vi "waitForCommandId.vi"(8 "error in (no error)":errorcluster, 11 "M1M3SAL in":refnum<class "M1M3SAL.lvclass">) -> (0 "error out":errorcluster, 2 "CommandId":T1, 3 "M1M3SAL out":refnum<class "M1M3SAL.lvclass">)   [LabVIEW 2016, in "M1M3SupportCommunicator.lvlib" / "M1M3SAL.lvclass"]
uses:
  M1M3SAL.lvclass
  DataTypes/Topics/Parts/CommandId.ctl
  M1M3SAL.lvclass/M1M3SAL.ctl
  UserEvents/UserEvents.lvclass/UserEvents.ctl
  UserEvents/UserEvents.lvclass
  DataTypes/Topics/M1M3SupportTopics.lvlib
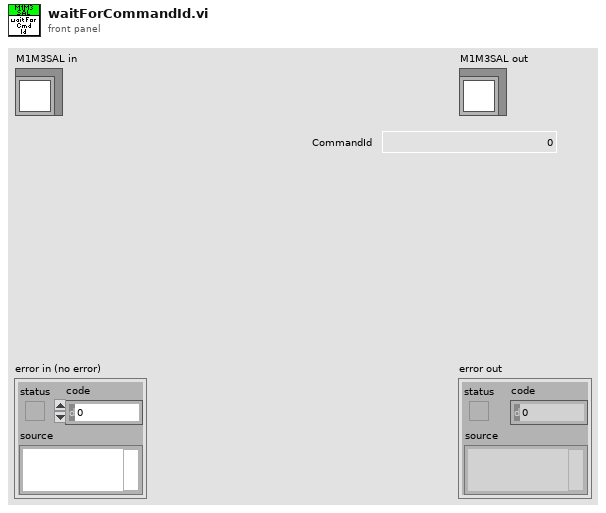
[diagram p1: front panel]
types:
  T1 = typedef "M1M3SupportTopics.lvlib/CommandId.ctl" = i32
  T2 = typedef "M1M3Communicator.lvlib/CommandId.ctl" = i32
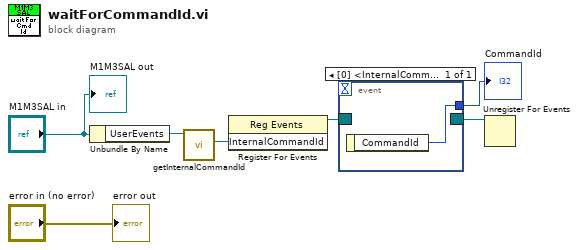
[diagram p0: block diagram]
diagram:
  n1 = Unbundle By Name("M1M3SAL in") -> ("UserEvents"=w7:refnum<class "UserEvents.lvclass">)
  n2 = call "getInternalCommandId.vi"("UserEvents in"=w7) -> ("InternalCommandId"=w6:refnum<user-event>)  [unwired: 9 in, 1 out]
  n3 = register-events(w6) -> (reference out=w5:refnum<event-registration>)  [unwired: 2 in, 1 out]
  n4 = event shown="[0] <InternalCommandId>: User Event" {
    selector: w5 -> [_]
    dyn-events: [_] -> w4
    timeout: _ -> [_]
    tunnel: [w8] -> w3
    event User Event {
      n5 = event-data() -> ("CommandId"=w8:T2)  [unwired: 1 in]
    }
  }
  "CommandId" <- w3
  n6 = Unregister For Events(event registration refnum=w4) -> ()  [unwired: 1 in, 1 out]
  "error out" <- "error in (no error)"
  "M1M3SAL out" <- "M1M3SAL in"
